vi "[MDI] Child Set Parent.vi"(8 "error in (no error)":errorcluster, 9 "child":refnum<vi>, 10 "child name":string, 11 "Interface of [MDI] Child in":refnum<class "Interface of [MDI] Child.lvclass">) -> (0 "error out":errorcluster, 3 "Interface of [MDI] Child out":refnum<class "Interface of [MDI] Child.lvclass">)   [LabVIEW 2020, in "[MDI] Child.lvlib" / "Interface of [MDI] Child.lvclass"]
uses:
  Interface of [MDI] Child.lvclass
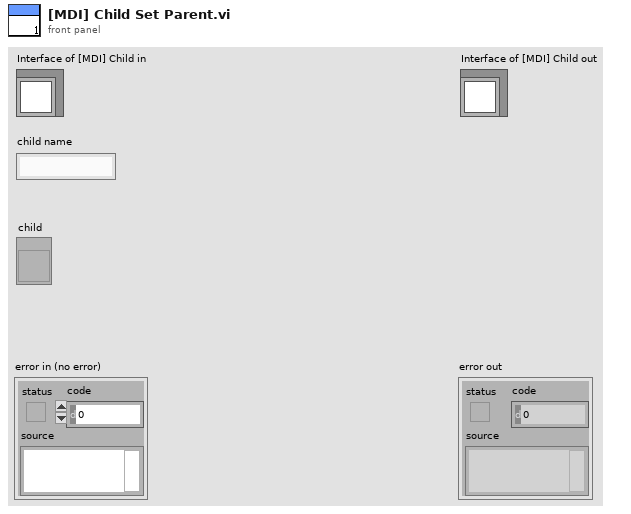
[diagram p1: front panel]
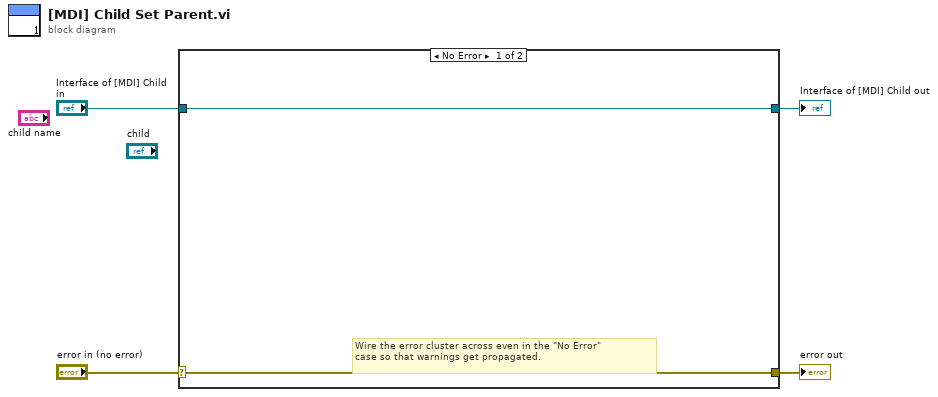
[diagram p0: block diagram]
diagram:
  n1 = case shown="No Error" "error in (no error)" {
    selector: "error in (no error)" -> [w5 w8]
    tunnel: [w5 w8] -> w3
    tunnel: [w6 w7] -> w1
    tunnel: "Interface of [MDI] Child in" -> [w6 w7]
    frame No Error {
      # "Wire the error cluster across even in the \"No Error\"\ncase so that warnings get propagated."
    }
    frame Error {
    }
  }
  "error out" <- w3
  "Interface of [MDI] Child out" <- w1
